vi "Init.vi"() -> (4 "a_hDevice":i32, 8 "Available":bool)   [LabVIEW 2016]
panel:
  out "NrOfDevices":i32
  out "Table":string[][](table)
  out "Info":string
  # "Avantes\nSolutions in Spectroscopy"
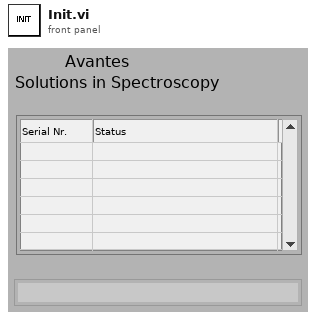
[diagram p1: front panel]
types:
  T1 = typedef "LVRowAndColumnTypeDef.ctl" = cluster{"Row":i32, "Column":i32}
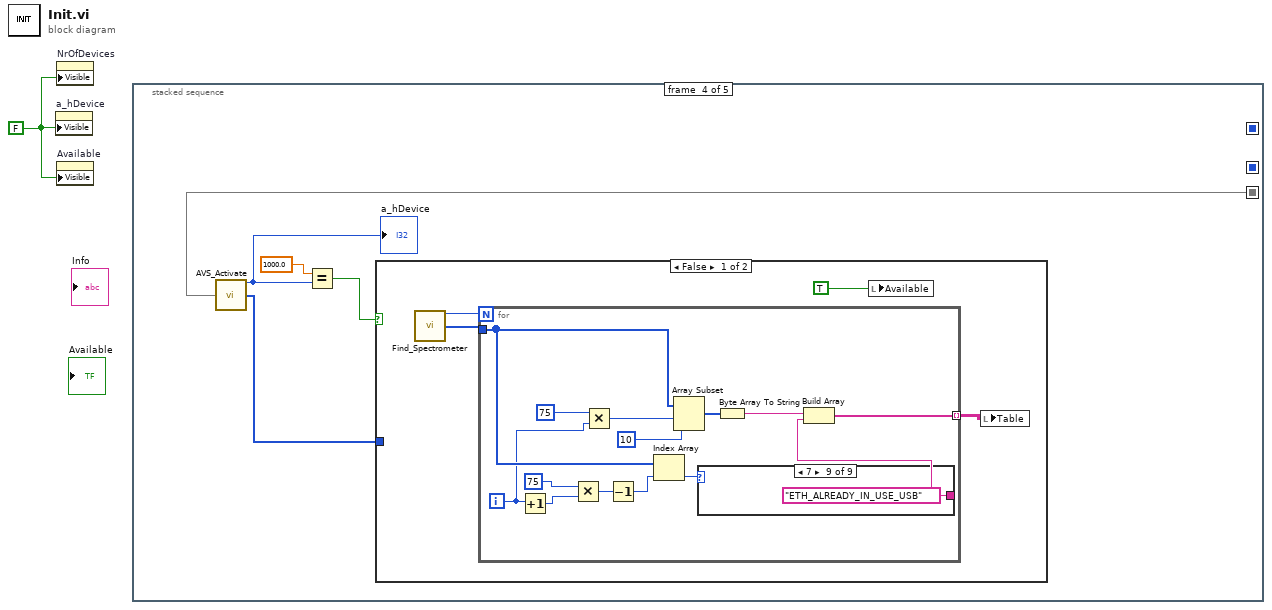
[diagram p0: block diagram]
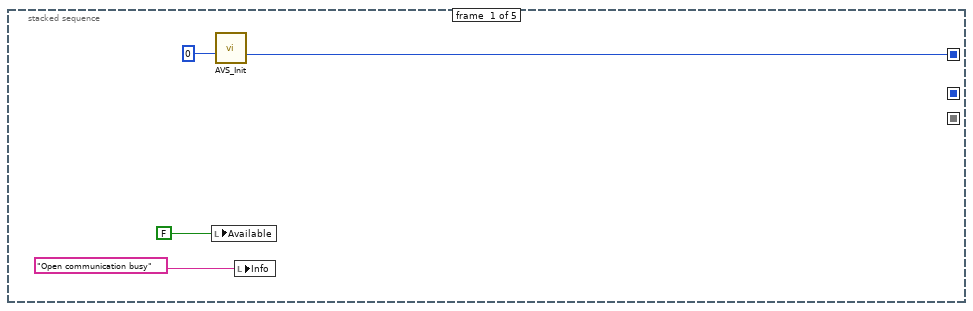
[diagram p2: hidden frame]
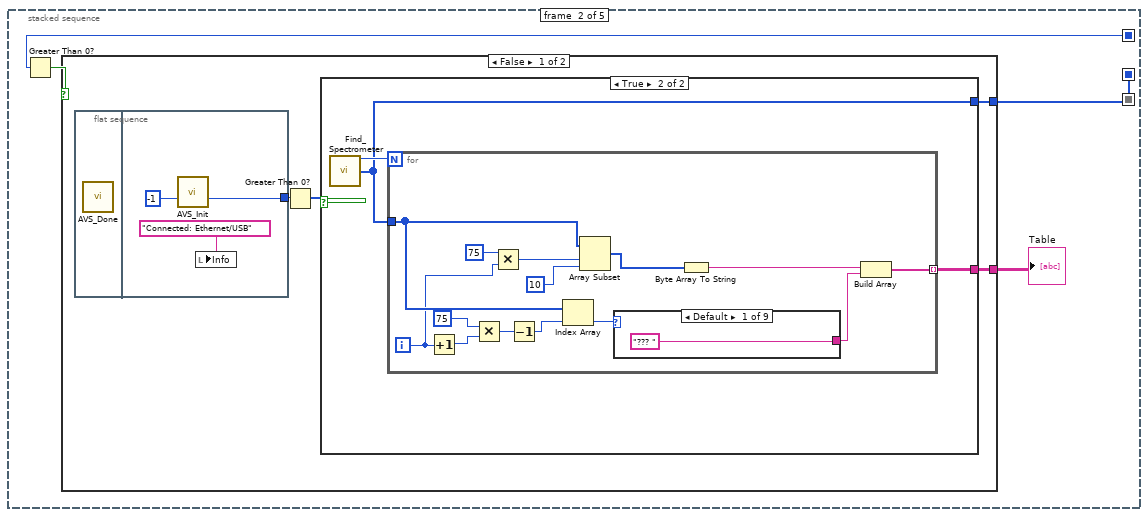
[diagram p3: hidden frame]
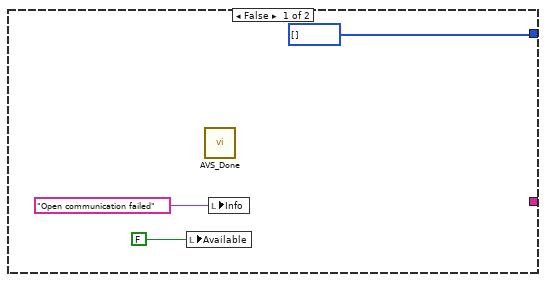
[diagram p4: hidden frame]
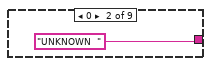
[diagram p5: hidden frame]
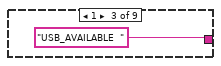
[diagram p6: hidden frame]
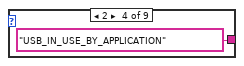
[diagram p7: hidden frame]
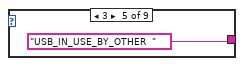
[diagram p8: hidden frame]
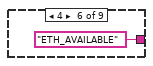
[diagram p9: hidden frame]
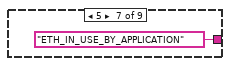
[diagram p10: hidden frame]
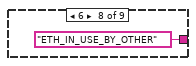
[diagram p11: hidden frame]
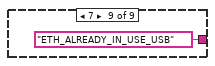
[diagram p12: hidden frame]
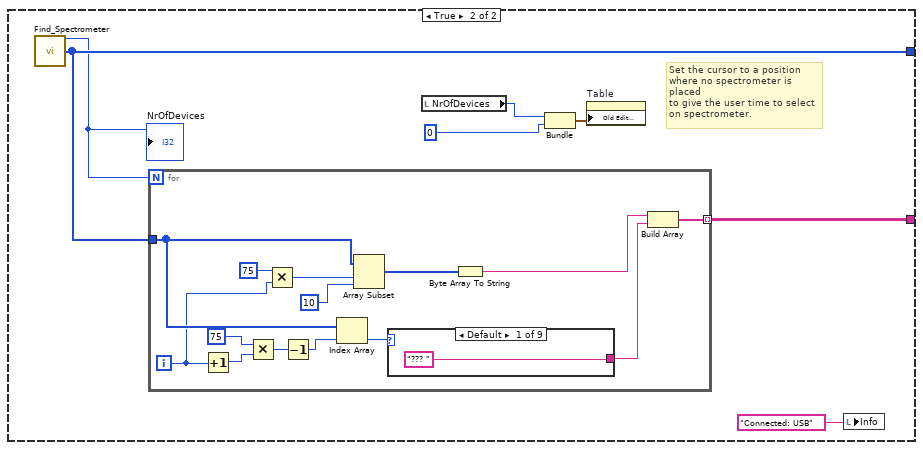
[diagram p13: hidden frame]
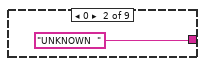
[diagram p14: hidden frame]
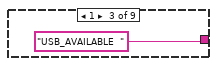
[diagram p15: hidden frame]
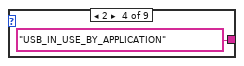
[diagram p16: hidden frame]
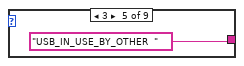
[diagram p17: hidden frame]
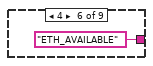
[diagram p18: hidden frame]
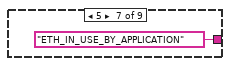
[diagram p19: hidden frame]
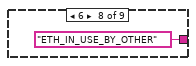
[diagram p20: hidden frame]
diagram:
  w1 = FALSE
  n1 = property on="a_hDevice" class="DigNum (strict)"("Visible"=w1) -> ()  [unwired: 2 in, 2 out]
  n2 = property on="NrOfDevices" class="DigNum (strict)"("Visible"=w1) -> ()  [unwired: 2 in, 2 out]
  n3 = property on="Available" class="Bool (strict)"("Visible"=w1) -> ()  [unwired: 2 in, 2 out]
  n4 = stacked-sequence {
    seq-local: [w3 _ _ _ _] -> [_ w8 _ _ _]
    seq-local: [_ w7 _ _ _] -> [_ _ w81 _ _]
    seq-local: [_ _ w78 _ _] -> [_ _ _ w90 _]
    frame #0 {
      n5 = local write "Available"(FALSE) -> ()
      n6 = call "AVS_Init.vi"("a_Port"=0) -> ("Output Value"=w3:i32)  [unwired: 14 in]
      n7 = local write "Info"("Open communication busy") -> ()
    }
    frame #1 {
      n8 = Greater Than 0?(x=w8) -> (x > 0?=w9:bool)
      n9 = case shown="False" w9 {
        tunnel: [w11 w51] -> w7
        tunnel: [w10 w46] -> w6
        frame False {
          n10 = flat-sequence {
            tunnel: [w44] -> w13
            frame #0 {
              n11 = call "AVS_Done.vi"() -> ()  [unwired: 19 in, 1 out]
            }
            frame #1 {
              n12 = call "AVS_Init.vi"("a_Port"=-1) -> ("Output Value"=w44:i32)  [unwired: 14 in]
              n13 = local write "Info"("Connected: Ethernet/USB") -> ()
            }
          }
          n14 = Greater Than 0?(x=w13) -> (x > 0?=w12:bool)
          n15 = case shown="True" w12 {
            tunnel: [u8[] [] ("List Output") w18] -> w11
            tunnel: [_ w17] -> w10
            frame False {
              n16 = local write "Available"(FALSE) -> ()
              n17 = call "AVS_Done.vi"() -> ()  [unwired: 19 in, 1 out]
              n18 = local write "Info"("Open communication failed") -> ()
            }
            frame True {
              n19 = call "Find_Spectrometer.vi"() -> ("NrOfDevices"=w19:i32, "AviableSpec"=w18:u8[])  [unwired: 14 in]
              n20 = for {
                N: w19 -> [_]
                tunnel: w18 -> [w25]
                tunnel: [w27] -> w17 mode=indexing
                i -> [w23]
                n21 = Increment(x=w23) -> (x+1=w22:i32)
                n22 = Multiply(x=75, y=w22) -> (x*y=w21:i32)
                n23 = Multiply(x=75, y=w23) -> (x*y=w29:i32)
                n24 = Decrement(x=w21) -> (x-1=w20:i32)
                n25 = Index Array(array=w25, index=w20) -> (element=w32:u8)
                n26 = Array Subset(array=w25, index=w29, length=10) -> (w24:u8[])
                n27 = case shown="Default" w32 {
                  tunnel: ["??? " "UNKNOWN  " "USB_AVAILABLE  " "USB_IN_USE_BY_APPLICATION" "USB_IN_USE_BY_OTHER  " "ETH_AVAILABLE" "ETH_IN_USE_BY_APPLICATION" "ETH_IN_USE_BY_OTHER" "ETH_ALREADY_IN_USE_USB"] -> w28
                  frame Default {
                  }
                  frame 0 {
                  }
                  frame 1 {
                  }
                  frame 2 {
                  }
                  frame 3 {
                  }
                  frame 4 {
                  }
                  frame 5 {
                  }
                  frame 6 {
                  }
                  frame 7 {
                  }
                }
                n28 = Byte Array To String(unsigned byte array=w24) -> (string=w26:string)
                n29 = Build Array(w26, w28) -> (w27:string[])
              }
            }
          }
        }
        frame True {
          # "Set the cursor to a position\nwhere no spectrometer is placed\nto give the user time to select\non spectrometer."
          n30 = call "Find_Spectrometer.vi"() -> ("NrOfDevices"=w50:i32, "AviableSpec"=w51:u8[])  [unwired: 14 in]
          "NrOfDevices" <- w50
          n31 = for {
            N: w50 -> [_]
            tunnel: w51 -> [w58]
            tunnel: [w60] -> w46 mode=indexing
            i -> [w56]
            n32 = Increment(x=w56) -> (x+1=w55:i32)
            n33 = Multiply(x=75, y=w55) -> (x*y=w54:i32)
            n34 = Multiply(x=75, y=w56) -> (x*y=w62:i32)
            n35 = Decrement(x=w54) -> (x-1=w53:i32)
            n36 = Index Array(array=w58, index=w53) -> (element=w65:u8)
            n37 = Array Subset(array=w58, index=w62, length=10) -> (w57:u8[])
            n38 = case shown="Default" w65 {
              tunnel: ["??? " "UNKNOWN  " "USB_AVAILABLE  " "USB_IN_USE_BY_APPLICATION" "USB_IN_USE_BY_OTHER  " "ETH_AVAILABLE" "ETH_IN_USE_BY_APPLICATION" "ETH_IN_USE_BY_OTHER" "ETH_ALREADY_IN_USE_USB "] -> w61
              frame Default {
              }
              frame 0 {
              }
              frame 1 {
              }
              frame 2 {
              }
              frame 3 {
              }
              frame 4 {
              }
              frame 5 {
              }
              frame 6 {
              }
              frame 7 {
              }
            }
            n39 = Byte Array To String(unsigned byte array=w57) -> (string=w59:string)
            n40 = Build Array(w59, w61) -> (w60:string[])
          }
          n41 = local read "NrOfDevices"() -> (w48:i32)
          n42 = Bundle("NrOfDevices"=w48, 0) -> (w49:cluster{" NrOfDevices":i32, i32})  [unwired: 1 in]
          n43 = property on="Table" class="Tbl (strict)"("Old Edit Position"=w49) -> ()  [unwired: 2 in, 2 out]
          n44 = local write "Info"("Connected: USB") -> ()
        }
      }
      "Table" <- w6
    }
    frame #2 {
      # "By clicking on the desired spectrometer the while loop is stopped \nand the spectrometer will be activated.\n\nNote: In this application you can activate just one spectrometer, if you want activate more start\nwith the sequence number 1 of this Stacked Sequence Structure again."
      n45 = local read "NrOfDevices"() -> (w77:i32)
      n46 = while {
        tunnel: w77 -> [w83]
        tunnel: [w86] -> w76
        stop <- w85 stop-if-true
        n47 = property on="Table" class="Tbl (strict)"() -> ("Old Edit Position"=w87:T1)  [unwired: 2 in, 2 out]
        n48 = Wait Until Next ms Multiple(millisecond multiple=u32 20) -> ()  [unwired: 1 out]
        n49 = Decrement(x=w83) -> (x-1=w84:i32)
        n50 = Unbundle(w87) -> ("Row"=w86:i32)  [unwired: 1 out]
        n51 = Less Or Equal?(x=w86, y=w84) -> (x <= y?=w85:bool)
      }
      n52 = Multiply(x=w76, y=75 ("x")) -> (x*y=w79:i32)
      n53 = Array Subset(array=w81, index=w79, length=75 ("x")) -> (w78:u8[])
    }
    frame #3 {
      n54 = call "AVS_Activate.vi"("a_pDeviceId"=w90) -> ("Output Value"=w91:i32, "a_pDeviceId"=w89:u8[])  [unwired: 13 in]
      "a_hDevice" <- w91
      n55 = Equal?(x=1000.0, y=w91) -> (x = y?=w93:bool)
      n56 = case shown="False" w93 {
        tunnel: w89 -> [_ w125]
        frame False {
          n57 = call "Find_Spectrometer.vi"() -> ("NrOfDevices"=w96:i32, "AviableSpec"=w97:u8[])  [unwired: 14 in]
          n58 = for {
            N: w96 -> [_]
            tunnel: w97 -> [w103]
            tunnel: [w105] -> w94 mode=indexing
            i -> [w101]
            n59 = Increment(x=w101) -> (x+1=w100:i32)
            n60 = Multiply(x=75, y=w100) -> (x*y=w99:i32)
            n61 = Multiply(x=75, y=w101) -> (x*y=w107:i32)
            n62 = Decrement(x=w99) -> (x-1=w98:i32)
            n63 = Index Array(array=w103, index=w98) -> (element=w110:u8)
            n64 = Array Subset(array=w103, index=w107, length=10) -> (w102:u8[])
            n65 = case shown="7" w110 {
              tunnel: ["??? " "UNKNOWN  " "USB_AVAILABLE  " "USB_IN_USE_BY_APPLICATION" "USB_IN_USE_BY_OTHER  " "ETH_AVAILABLE" "ETH_IN_USE_BY_APPLICATION" "ETH_IN_USE_BY_OTHER" "ETH_ALREADY_IN_USE_USB"] -> w106
              frame Default {
              }
              frame 0 {
              }
              frame 1 {
              }
              frame 2 {
              }
              frame 3 {
              }
              frame 4 {
              }
              frame 5 {
              }
              frame 6 {
              }
              frame 7 {
              }
            }
            n66 = Byte Array To String(unsigned byte array=w102) -> (string=w104:string)
            n67 = Build Array(w104, w106) -> (w105:string[])
          }
          n68 = local write "Available"(TRUE) -> ()
          n69 = local write "Table"(w94) -> ()
        }
        frame True {
          n70 = Array Subset(array=w125, index=0 ("length"), length=10) -> (w122:u8[])
          n71 = Byte Array To String(unsigned byte array=w122) -> (string=w124:string)
          n72 = Concatenate Strings("Error opening device", w124) -> (w127:string)
          n73 = local write "Info"(w127) -> ()
          n74 = local write "Available"(FALSE) -> ()
        }
      }
    }
    frame #4 {
      n75 = Wait (ms)(milliseconds to wait=u32 2000) -> ()  [unwired: 1 out]
    }
  }
